vi "pcgs_close_log.vi"(8 "error in (no error)":errorcluster, 11 "pcfs in":refnum<class "pcfs.lvclass">) -> (0 "error out":errorcluster, 3 "pcfs out":refnum<class "pcfs.lvclass">)   [LabVIEW 2015, in "pcfs.lvclass"]
uses:
  pcfs.lvclass
  pcfs.lvclass/pcfs.ctl
  Detector_Class/Picoquant/Picoquant_generic/picoquant_generic.lvclass
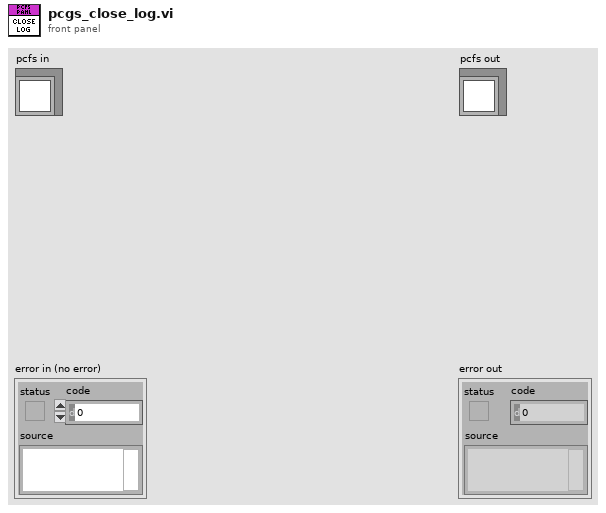
[diagram p1: front panel]
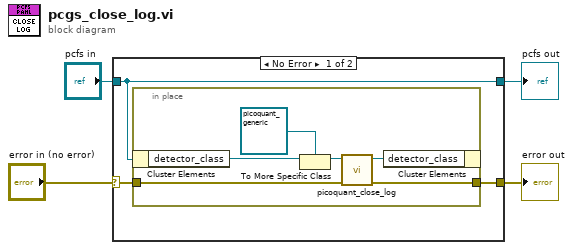
[diagram p0: block diagram]
diagram:
  n1 = case shown="No Error" "error in (no error)" {
    selector: "error in (no error)" -> [w6 w15]
    tunnel: [w5 w15] -> w3
    tunnel: [w7 w14] -> w1
    tunnel: "pcfs in" -> [w7 w14]
    frame No Error {
      n2 = in-place {
        in-place-border: w6 -> [w10]
        in-place-border: [w8] -> w5
        n3 = in-place-cluster #1(w7) -> ("detector_class"=w12:refnum<class "detector.lvclass">)
        n4 = To More Specific Class(target class=refnum<class "picoquant_generic.lvclass"> refnum ("picoquant_generic in"), reference=w12) -> (specific class reference=w11:refnum<class "picoquant_generic.lvclass">)  [unwired: 1 in, 1 out]
        n5 = call-dynamic "picoquant_close_log.vi"("error in (no error)"=w10, "picoquant_generic in"=w11) -> ("error out"=w8:errorcluster, "picoquant_generic out"=w9:refnum<class "picoquant_generic.lvclass">)  [unwired: 8 in]
        n6 = in-place-cluster #1("detector_class"=w9) -> ()  [unwired: 1 out]
      }
    }
    frame Error {
    }
  }
  "error out" <- w3
  "pcfs out" <- w1
